vi "F Dwf Digital In Trigger Match Set.vi"(6 "cBitStuffing":i32, 7 "fsValue":u32, 8 "error in (no error)":errorcluster, 9 "fsMask":u32, 10 "iPin":i32, 11 "hdwf":i32) -> (0 "error out":errorcluster, 3 "function return":i32)   [LabVIEW 2019, in "Olasdwf.lvlib"]
doc: "DWFAPI int FDwfDigitalInTriggerMatchSet(HDWF hdwf, int iPin, unsigned int fsMask, unsigned int fsValue, int cBitStuffing);"
uses:
  Olasdwf.lvlib
  Windows/System32/dwf.dll
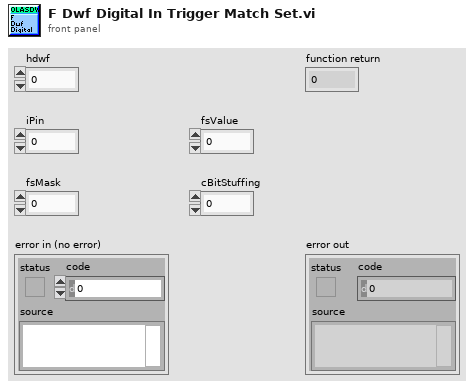
[diagram p1: front panel]
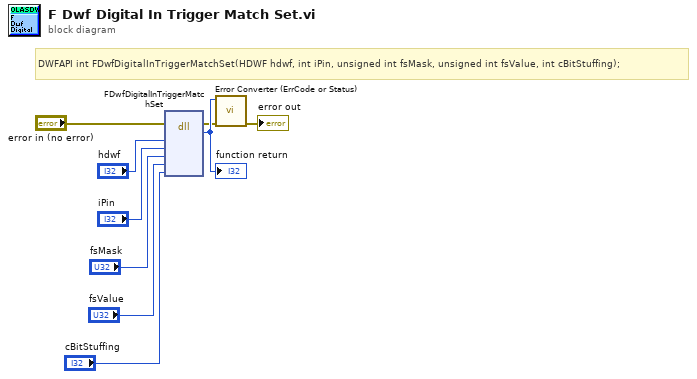
[diagram p0: block diagram]
diagram:
  # "DWFAPI int FDwfDigitalInTriggerMatchSet(HDWF hdwf, int iPin, unsigned int fsMask, unsigned int fsValue, int cBitStuffing);"
  n1 = dll-call lib="C:/Windows/System32/dwf.*" fn="FDwfDigitalInTriggerMatchSet"(error in="error in (no error)", "hdwf"="hdwf", "iPin"="iPin", "fsMask"="fsMask", "fsValue"="fsValue", "cBitStuffing"="cBitStuffing") -> (error out=w2:errorcluster, w9:i32)  [unwired: 7 in, 1 out]
  "function return" <- w9
  n2 = call "Error Converter (ErrCode or Status).vi"("error in (no error)"=w2, "error code"=w9) -> ("error out"=→"error out":errorcluster)  [unwired: 9 in]
